vi "Get All ECID Data.vi"(8 "error in (no error)":errorcluster) -> (0 "error out":errorcluster, 3 "ECID Data":T1[](array[typedef]))   [LabVIEW 2020, in "SECS Communication.lvlib" / "SECS Data Class.lvclass"]
uses:
  SECS Data Class.lvclass
  ECID Data.ctl
  SECS-II Class/Format Code.ctl
  SECS Data Class.lvclass/SECS Data Class.ctl
  SECS-II Class/SECS-II Class.lvclass
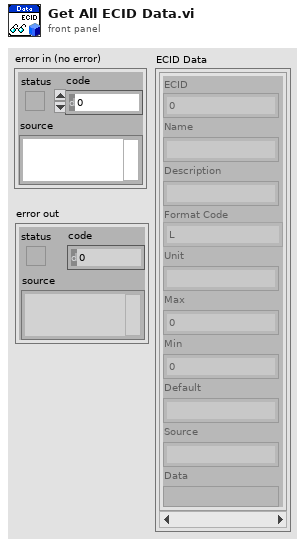
[diagram p1: front panel]
types:
  T1 = typedef "SECS Communication.lvlib/SECS Data Class.lvclass/ECID Data.ctl" = cluster{"ECID":u32, "Name":string, "Description":string, "Format Code":T2, "Unit":string, "Max":dbl, "Min":dbl, "Default":string, "Source":string, "Data":variant}
  T2 = typedef "SECS Communication.lvlib/SECS-II Class.lvclass/Format Code.ctl" = enum16{"L", "A", "B", "Boolean", "J", "I1", "I2", "I4", "I8", "U1", "U2", "U4", "U8", "F4", "F8", "Char"}
  T3 = typedef "SECS Data.lvlib/SECS Data Class.lvclass/ECID Data.ctl" = cluster{"ECID":u32, "Name":string, "Description":string, "Format Code":T2, "Unit":string, "Max":dbl, "Min":dbl, "Default":string, "Source":string, "Data":variant}
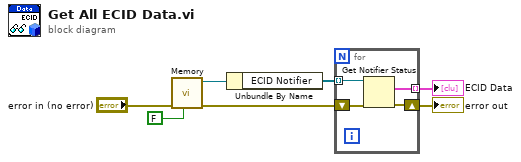
[diagram p0: block diagram]
diagram:
  n1 = call "Memory.vi"("Put"=FALSE, "error in (no error)"="error in (no error)") -> ("error out"=w4:errorcluster, "SECS Data Class out"=w5:refnum<class "SECS Data Class.lvclass">)  [unwired: 8 in]
  n2 = Unbundle By Name(w5) -> ("ECID Notifier"=w3:refnum<notifier>[])
  n3 = for {
    shift-right: [w9] -> w1
    shift-left: w4 -> [w10]
    tunnel: w3 -> [w11] mode=indexing
    tunnel: [w8] -> w2 mode=indexing
    n4 = Get Notifier Status(notifier=w11, error in (no error)=w10) -> (current notification=w8:T3, error out=w9:errorcluster)  [unwired: 3 out]
  }
  "error out" <- w1
  "ECID Data" <- w2
